vi "time-to-array.vi"(1 "Array":string[](array[string]), 2 "index":i32) -> (0 "output array":string[](array[string]))   [LabVIEW 2023]
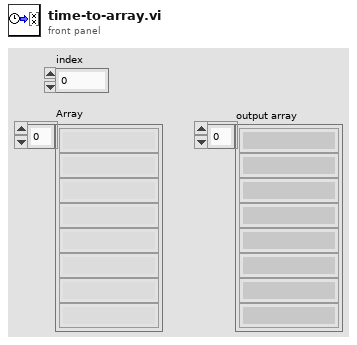
[diagram p1: front panel]
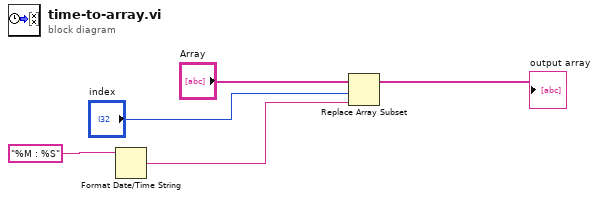
[diagram p0: block diagram]
diagram:
  n1 = Format Date/Time String(time format string (%c)="%M : %S") -> (date/time string=w3:string)  [unwired: 2 in]
  n2 = Replace Array Subset(array="Array", new element=w3, index="index") -> (→"output array":string[])
